vi "DAC Stop.vi"(8 "error in (no error)":errorcluster, 11 "DAC HeatFlow Load dU in":refnum<class "DAC HeatFlow Load dU.lvclass">) -> (0 "error out":errorcluster, 3 "DAC HeatFlow Load dU out":refnum<class "DAC HeatFlow Load dU.lvclass">)   [LabVIEW 2019, in "DAC.lvlib" / "DAC HeatFlow Load dU.lvclass"]
uses:
  DAC HeatFlow Load dU.lvclass
  C:/Users/krio/Documents/LV_Projects/test-stand/App/DAC/DAC.lvclass
  DAC.lvclass/DAC.ctl
  DAC HeatFlow Load dU.lvclass/DAC HeatFlow Load dU.ctl
  DAC.lvclass
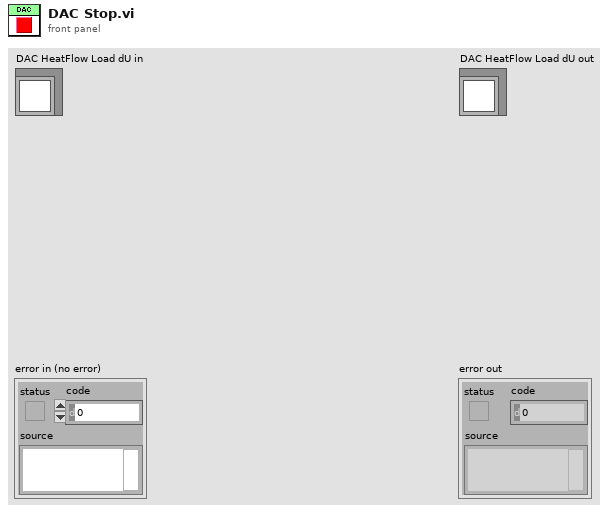
[diagram p1: front panel]
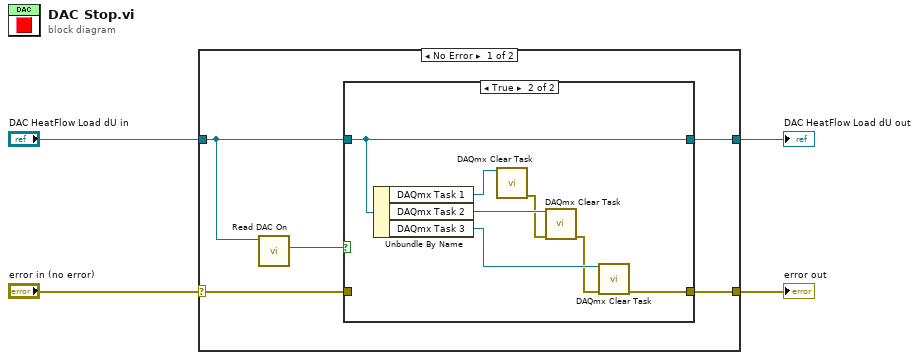
[diagram p0: block diagram]
diagram:
  n1 = case shown="No Error" "error in (no error)" {
    selector: "error in (no error)" -> [w6 w20]
    tunnel: [w5 w20] -> w1
    tunnel: [w7 w19] -> w3
    tunnel: "DAC HeatFlow Load dU in" -> [w9 w19]
    frame No Error {
      n2 = call "Read DAC On.vi"("DAC in"=w9) -> ("DAC On"=w8:bool)  [unwired: 8 in, 2 out]
      n3 = case shown="True" w8 {
        tunnel: w9 -> [w11 w18]
        tunnel: [w11 w18] -> w7
        tunnel: w6 -> [w10 _]
        tunnel: [w10 w12] -> w5
        frame False {
        }
        frame True {
          n4 = Unbundle By Name(w18) -> ("DAQmx Task 1"=w17:refnum<k21>, "DAQmx Task 2"=w16:refnum<k21>, "DAQmx Task 3"=w15:refnum<k21>)
          n5 = call <vilib>:"DAQmx Clear Task.vi"("task in"=w17) -> ("error out"=w14:errorcluster)  [unwired: 14 in]
          n6 = call <vilib>:"DAQmx Clear Task.vi"("task in"=w16, "error in"=w14) -> ("error out"=w13:errorcluster)  [unwired: 13 in]
          n7 = call <vilib>:"DAQmx Clear Task.vi"("task in"=w15, "error in"=w13) -> ("error out"=w12:errorcluster)  [unwired: 13 in]
        }
      }
    }
    frame Error {
    }
  }
  "error out" <- w1
  "DAC HeatFlow Load dU out" <- w3
